vi "Bai1_1.vi"() -> ()   [LabVIEW 2023]
panel:
  in  "stop":bool
  out "Can Divide":dbl
  out "Divide":dbl
  out "Multiple":dbl
  out "Subtraction":dbl
  out "Addition":dbl
  in  "y":dbl
  in  "x":dbl
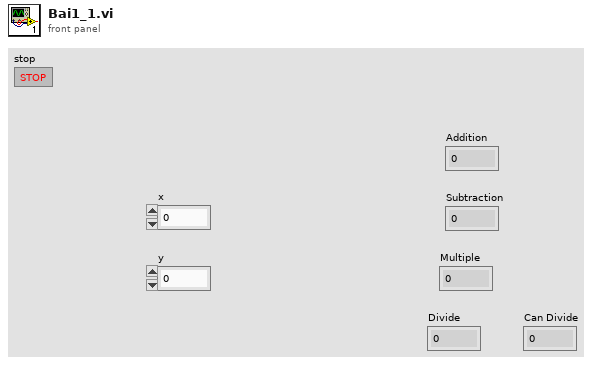
[diagram p1: front panel]
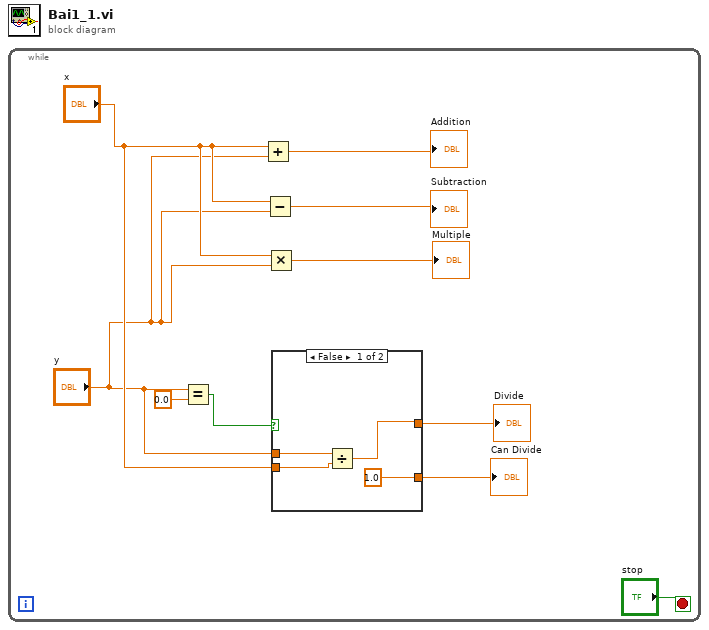
[diagram p0: block diagram]
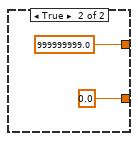
[diagram p2: hidden frame]
diagram:
  n1 = while {
    stop <- "stop" stop-if-true
    n2 = Equal?(x="y", y=0.0) -> (x = y?=w6:bool)
    n3 = Add(x="x", y="y") -> (x+y=→"Addition":dbl)
    n4 = Subtract(x="x", y="y") -> (x-y=→"Subtraction":dbl)
    n5 = Multiply(x="x", y="y") -> (x*y=→"Multiple":dbl)
    n6 = case shown="False" w6 {
      tunnel: "y" -> [w14 _]
      tunnel: "x" -> [w12 _]
      tunnel: [w11 999999999.0] -> w3
      tunnel: [1.0 0.0] -> w2
      frame False {
        n7 = Divide(x=w14, y=w12) -> (x/y=w11:dbl)
      }
      frame True {
      }
    }
    "Divide" <- w3
    "Can Divide" <- w2
  }
